vi "GetAppOutput.vi"(8 "error in (no error)":errorcluster, 11 "RingdownPlugin in":refnum<class "RingdownPlugin.lvclass">) -> (0 "error out":errorcluster, 3 "RingdownPlugin out":refnum<class "RingdownPlugin.lvclass">)   [LabVIEW 2017, in "AppPlugins.lvlib" / "RingdownPlugin.lvclass"]
uses:
  RingdownPlugin.lvclass
  C:/dev/Work/PARTF/Modules/AppPlugins/AppPluginBaseClass/AppPluginsBase.lvclass
  TypeDef/RingdownOutput.ctl
  RingdownPlugin.lvclass/RingdownPlugin.ctl
  Accessors/Read RingdownConfig.vi
  <vilib>/Utility/error.llb/Error Cluster From Error Code.vi
  <vilib>/ErrorRing/Error Ring.xnode
panel:
  out "Damping ratio":dbl[](array[numeric])
  out "Warning":i32
  out "Output Parameters":T1
  out "Time of process":dbl
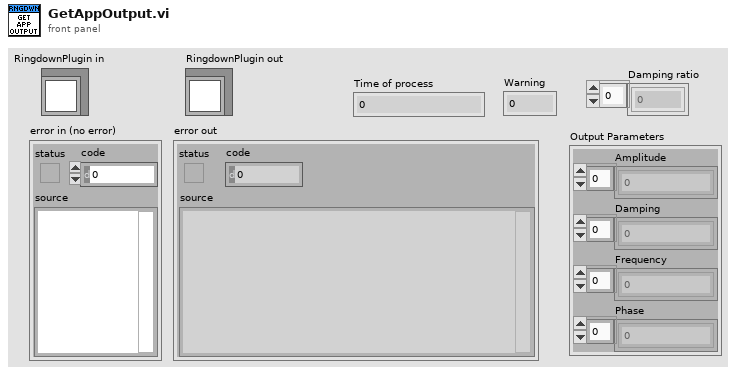
[diagram p1: front panel]
types:
  T1 = cluster{"Amplitude":dbl[], "Damping":dbl[], "Frequency":dbl[], "Phase":dbl[]}
  T2 = typedef "AppPlugins.lvlib/RingdownPlugin.lvclass/RingdownOutput.ctl" = cluster{"FramesPerSecond":dbl, "PronyEstimate":dbl[], "RingdownParameters":cluster{"Amplitude":dbl[], "Damping":dbl[], "Frequency":dbl[], "Phase":dbl[]}, "ReportingTime":dbl, "DataSize":u32, "InputSignal":dbl[]}
  T3 = typedef "AppPlugins.lvlib/RingdownPlugin.lvclass/RingdownConfig.ctl" = cluster{"Config":cluster{"Addmod":i32, "Scalmod":i32, "Lpocon":i32, "Pircon":i32, "Dmodes":i32, "Lpmcon":u16, "Lpacon":u16, "Fbcon":u16, "Ordcon":i32, "Trimre":dbl, "Ftrimh":dbl, "Ftriml":dbl}, "Window":cluster{"StOffset":i32, "EndOffset":i32, "Length":i32}, "V index":i32, "I index":i32, "PosSeq":bool}
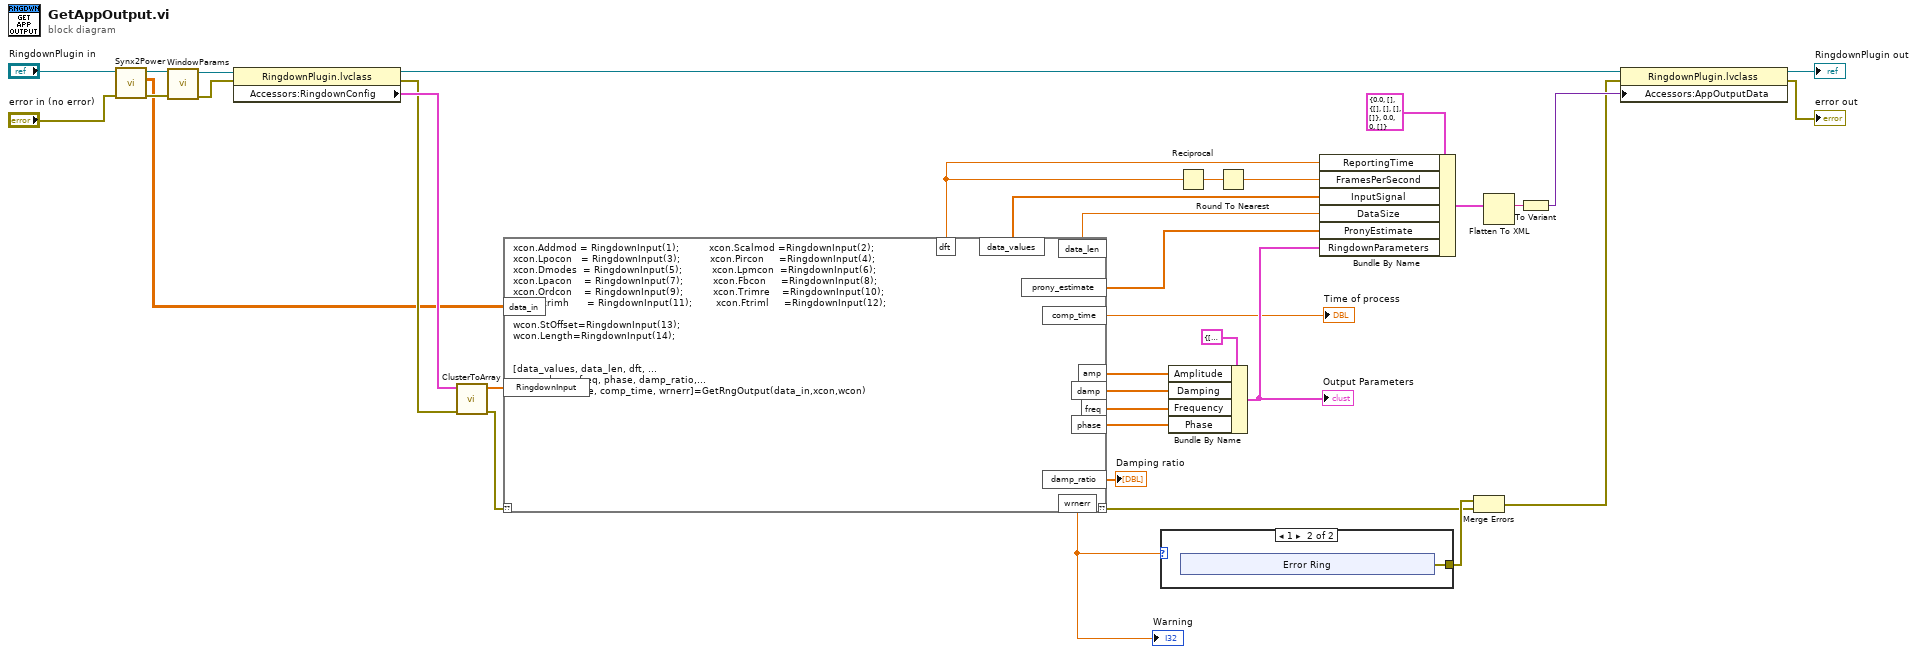
[diagram p0: block diagram]
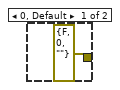
[diagram p2: hidden frame]
diagram:
  n1 = call "Synx2Power.vi"("error in (no error)"="error in (no error)", "RingdownPlugin in"="RingdownPlugin in") -> ("error out"=w29:errorcluster, "Active Power"=w11:dbl[][], "RingdownPlugin out"=w28:refnum<class "RingdownPlugin.lvclass">)  [unwired: 6 in, 1 out]
  n2 = call "WindowParams.vi"("error in (no error)"=w29, "RingdownPlugin"=w28) -> ("error out"=w26:errorcluster, "RingdownPlugin.lvclass"=w27:refnum<class "RingdownPlugin.lvclass">)  [unwired: 8 in]
  n3 = property class="RingdownPlugin.lvclass"(reference=w27, error in=w26) -> (reference out=w25:refnum<class "RingdownPlugin.lvclass">, error out=w17:errorcluster, "Accessors:RingdownConfig"=w18:T3)
  n4 = call "ClusterToArray.vi"("error in (no error)"=w17, "RingdownConfig"=w18) -> ("error out"=w16:errorcluster, "RingdownInput"=w10:dbl[])  [unwired: 8 in]
  n5 = script code="xcon.Addmod = RingdownInput(1);          xcon.Scalmod =RingdownInput(2);        \nxcon.Lpocon   = RingdownInput(3);          xcon.Pircon     =RingdownInput(4);             \nxcon.Dmodes  = RingdownInput(5);          xcon.Lpmcon  =RingdownInput(6); \nxcon.Lpacon    = RingdownInput(7);          xcon.Fbcon     =RingdownInput(8);     \nxcon.Ordcon    = RingdownInput(9);          xcon.Trimre    =RingdownInput(10);          \nxcon.Ftrimh      = RingdownInput(11);        xcon.Ftriml     =RingdownInput(12); \n\nwcon.StOffset=RingdownInput(13);           \nwcon.Length=RingdownInput(14);  \n\n\n[data_values, data_len, dft, ...\n  amp, damp, freq, phase, damp_ratio,...\n  prony_estimate, comp_time, wrnerr]=GetRngOutput(data_in,xcon,wcon)"("??"=w16, "data_in"=w11, "RingdownInput"=w10) -> ("??"=w3:errorcluster, "dft"=w23:dbl, "data_values"=w22:dbl[], "data_len"=w21:dbl, "prony_estimate"=w20:dbl[], "comp_time"=→"Time of process":dbl, "amp"=w15:dbl[], "damp"=w14:dbl[], "freq"=w13:dbl[], "phase"=w12:dbl[], "damp_ratio"=→"Damping ratio":dbl[], "wrnerr"=w1:dbl)
  "Warning" <- w1
  n6 = case shown="1" w1 {
    tunnel: [errorcluster {"status"=FALSE, "code"=0, "source"=""} ("error out") w38] -> w4
    frame 0, Default {
    }
    frame 1 {
      n7 = xnode "Error Ring"() -> ("error out"=w38:errorcluster)
    }
  }
  n8 = Bundle By Name(cluster=T1 {"Amplitude"=[], "Damping"=[], "Frequency"=[], "Phase"=[0.0, 0.0, 0.0, 0.0, 0.0, 0.0, 0.0, 0.0, 0.0, 0.0, 0.0, 0.0, 0.0, 0.0, 0.0, 0.0]} ("RingdownParameters"), "Amplitude"=w15, "Damping"=w14, "Frequency"=w13, "Phase"=w12) -> (w24:T1)
  "Output Parameters" <- w24
  n9 = Reciprocal(x=w23) -> (1/x=w34:dbl)
  n10 = Round To Nearest(number=w34) -> (nearest integer value=w33:dbl)
  n11 = Bundle By Name(cluster=T2 {"FramesPerSecond"=0.0, "PronyEstimate"=[], "RingdownParameters"={"Amplitude"=[], "Damping"=[], "Frequency"=[], "Phase"=[]}, "ReportingTime"=0.0, "DataSize"=0, "InputSignal"=[]} ("RingdownOutput"), "ReportingTime"=w23, "FramesPerSecond"=w33, "InputSignal"=w22, "DataSize"=w21, "PronyEstimate"=w20, "RingdownParameters"=w24) -> (w8:T2)
  n12 = Merge Errors(w4, w3) -> (w2:errorcluster)
  n13 = Flatten To XML(anything=w8) -> (xml string=w7:string)
  n14 = To Variant(anything=w7) -> (Variant=w6:variant)
  n15 = property class="RingdownPlugin.lvclass"(reference=w25, error in=w2, "Accessors:AppOutputData"=w6) -> (reference out=→"RingdownPlugin out":refnum<class "RingdownPlugin.lvclass">, error out=→"error out":errorcluster)
